vi "Convert Filter to INI String.vi"(11 "Filter Info":T1={"Filter Column"=enum."Description", "Filter Type"=enum."Contains", "Filter Value"="", "New Data?"=FALSE, "Case Sensitive?"=FALSE, "Enabled?"=FALSE}) -> (3 "INI String":string)   [LabVIEW 2020, in "VI Properties Editor.lvlib"]
doc: "Converts <B>Filter Info</B> to an INI string to be stored."
uses:
  VI Properties Editor.lvlib
  CTLs/Column Name.ctl
  CTLs/Filter Type.ctl
  CTLs/Filter Info.ctl
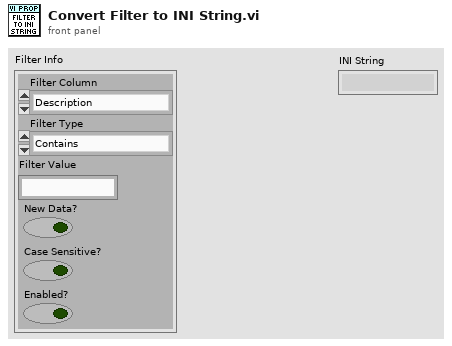
[diagram p1: front panel]
types:
  T1 = typedef "VI Properties Editor.lvlib/Filter Info.ctl" = cluster{"Filter Column":T2, "Filter Type":T3, "Filter Value":string, "New Data?":bool, "Case Sensitive?":bool, "Enabled?":bool}
  T2 = typedef "VI Properties Editor.lvlib/Column Name.ctl" = enum16{"Name", "Path", "Type", "Window Title", "Description", "Help Path", "Help Tag", "Custom Title?", "Reentrancy", "Inlined?", "Help URL", "Help Type", "Allow Debugging?", "Auto Error Handling?", "Run When Opened?", "Suspend When Called?", "Priority", "Preferred Exec Sytem", "Control Label", "Control Caption", "Control Description", "Control Tip Strip"}
  T3 = typedef "VI Properties Editor.lvlib/Filter Type.ctl" = enum16{"Contains", "Equals", "Starts with", "Ends with", "Is empty", "Does not contain", "Does not equal", "Is not empty"}
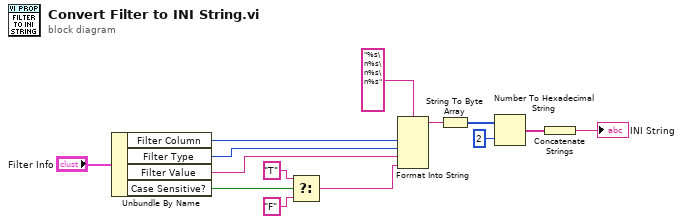
[diagram p0: block diagram]
diagram:
  n1 = Unbundle By Name("Filter Info") -> ("Filter Column"=w11:T2, "Filter Type"=w10:T3, "Filter Value"=w9:string, "Case Sensitive?"=w4:bool)
  n2 = Select(t="T", s=w4, f="F") -> (s? t:f=w1:string)
  n3 = Format Into String(format string="%s\n%s\n%s\n%s", w11, w10, w9, w1) -> (resulting string=w8:string)  [unwired: 2 in, 1 out]
  n4 = String To Byte Array(string=w8) -> (unsigned byte array=w13:u8[])
  n5 = Number To Hexadecimal String(1:i16 2 ("width (-)"), 2:w13) -> (0:w7:string[])
  n6 = Concatenate Strings(w7) -> (→"INI String":string)
